vi "PI Controller.vi"(0 "Ts [s]":dbl, 1 "u_max":dbl caption="Maximum Control Signal [V]", 5 "Kp":dbl, 7 "Ti [s]":dbl, 9 "Reference Value":dbl, 11 "Process Value":dbl, 12 "u_min":dbl caption="Minimum Control Signal [V]") -> (8 "Output":dbl)   [LabVIEW 2022 SP3]
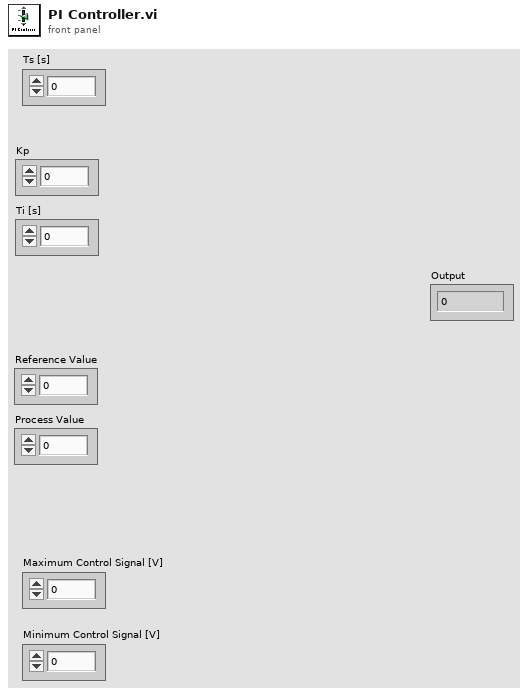
[diagram p1: front panel]
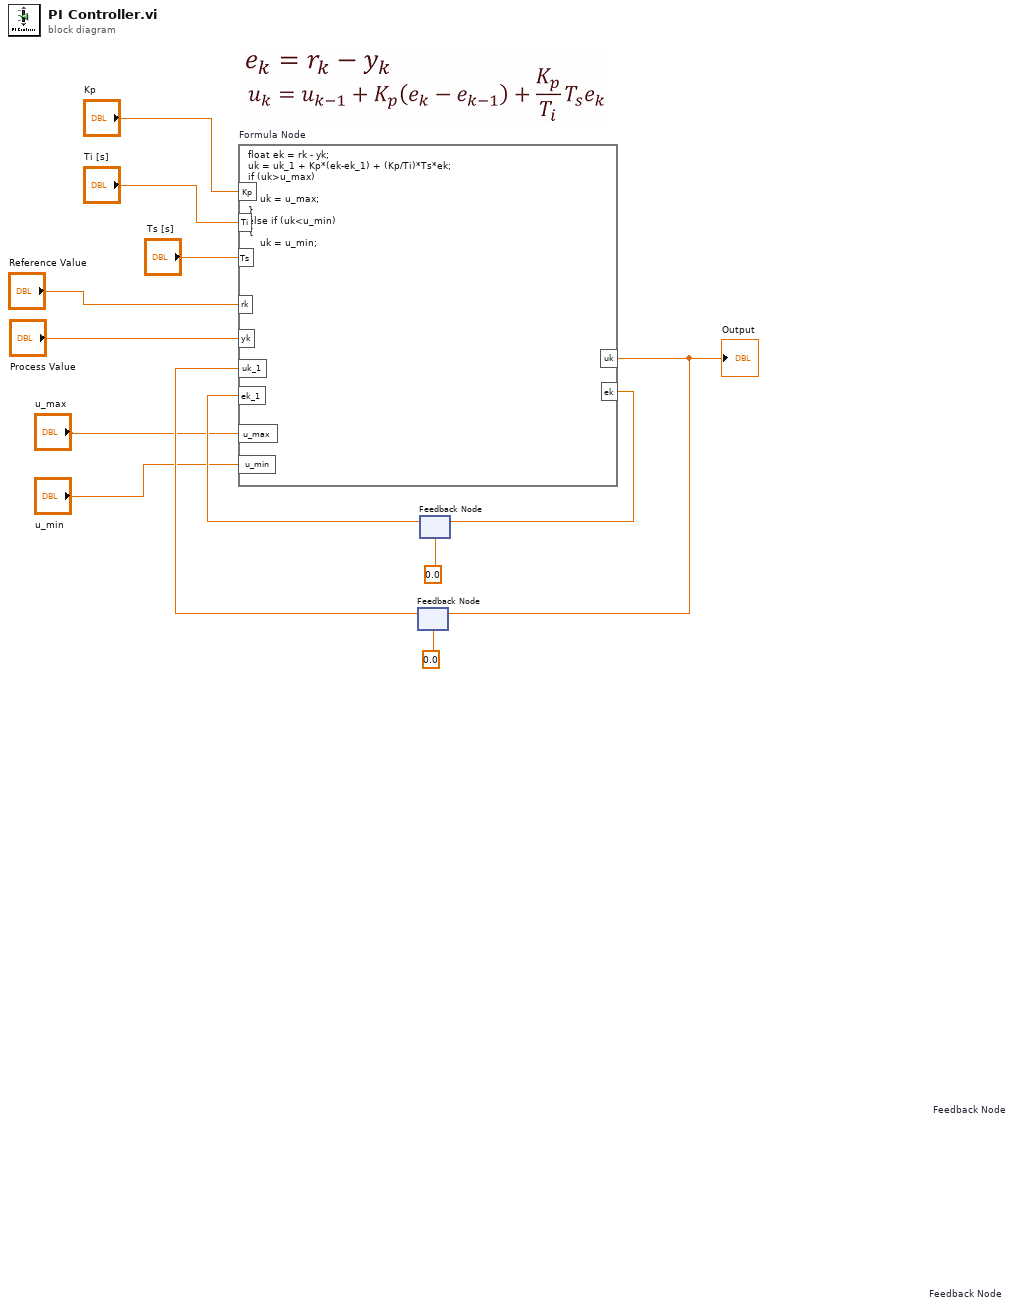
[diagram p0: block diagram]
diagram:
  n1 = feedback #1 "Feedback Node"(0.0 ("uk")) -> (w9:dbl)
  n2 = feedback #2 "Feedback Node"(0.0) -> (w11:dbl)
  n3 = formula code="float ek = rk - yk;\nuk = uk_1 + Kp*(ek-ek_1) + (Kp/Ti)*Ts*ek;\nif (uk>u_max)\n{\n    uk = u_max;\n}\nelse if (uk<u_min)\n{\n    uk = u_min;\n}"("rk"="Reference Value", "yk"="Process Value", "uk_1"=w9, "Ti"="Ti [s]", "Kp"="Kp", "Ts"="Ts [s]", "ek_1"=w11, "u_max"="u_max", "u_min"="u_min") -> ("uk"=w10:dbl, "ek"=w12:dbl)
  "Output" <- w10
  n4 = feedback-in #1(w10) -> ()
  n5 = feedback-in #2(w12) -> ()
